vi "PH_Trendviewer_Powermeter.add new result.vi"(0 "i ref in":refnum<vi>, 2 "Energy [J]":dbl, 5 "error in (no error)":errorcluster) -> (14 "i ref out":refnum<vi>, 19 "error out":errorcluster)   [LabVIEW 2014, in "PH_Trendviewer_Powermeter.lvlib"]
doc: "This VI investigates the new incoming data and adds them to the results already collected."
uses:
  PH_Trendviewer_Powermeter.lvlib
  PH_Common/PH_Common.lvlib
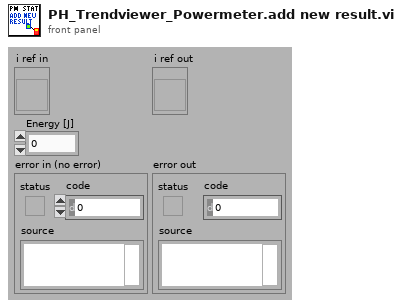
[diagram p1: front panel]
types:
  T1 = cluster{"Time Stamp":timestamp, "Energy [J]":dbl}
  T2 = typedef "PH_Trendviewer_Powermeter.lvlib/PH_Trendviewer_Powermeter.i attribute.ctl" = cluster{"GUI Refs ":cluster{"Status":refnum<vi>, "Result Graph":refnum<vi>, "Mean Data":refnum<vi>, "Std Dev Data":refnum<vi>, "Dummy Mean":refnum<vi>, "Dummy Std Dev":refnum<vi>, "Export Data":refnum<vi>, "Stat or Trend":refnum<vi>, "Delete":refnum<vi>, "Powermeter":refnum<vi>, "Start":refnum<vi>}, "Powermeter":string, "Stat or Trend":bool, "Start":bool, "Data":cluster{"Time Stamp":timestamp, "Energy [J]":dbl}[], "Datasets strored":i32, "Dataarray Size":i32}
  T3 = cluster{"Time Stamp":timestamp, "Energy [J]":dbl}[]
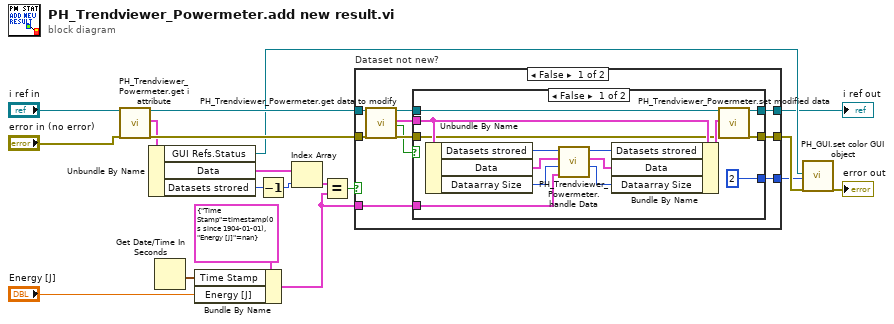
[diagram p0: block diagram]
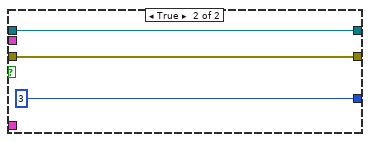
[diagram p2: hidden frame]
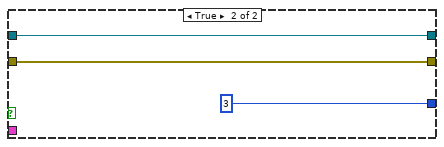
[diagram p3: hidden frame]
diagram:
  n1 = call "PH_Trendviewer_Powermeter.get i attribute.vi"("i ref in"="i ref in", "error in (no error)"="error in (no error)") -> ("i ref out"=w15:refnum<vi>, "i attribute"=w14:T2, "error out"=w16:errorcluster)  [unwired: 15 in]
  n2 = Unbundle By Name(w14) -> ("GUI Refs.Status"=w12:refnum<vi>, "Data"=w8:T3, "Datasets strored"=w6:i32)
  n3 = Get Date/Time In Seconds() -> (seconds since 1Jan1904=w18:timestamp)
  n4 = Bundle By Name(cluster=T1 {"Time Stamp"=timestamp(0 s since 1904-01-01), "Energy [J]"=nan} ("Dataset"), "Time Stamp"=w18, "Energy [J]"="Energy [J]") -> (w1:T1)
  n5 = Decrement(x=w6) -> (x-1=w9:i32)
  n6 = Index Array(array=w8, index=w9) -> (element=w10:T1)
  n7 = Equal?(x=w10, y=w1) -> (x = y?=w7:bool)
  n8 = case "Dataset not new?" shown="False" w7 {
    tunnel: [w26 w49] -> w3
    tunnel: w16 -> [w24 w48]
    tunnel: w15 -> [w23 w49]
    tunnel: [w22 w48] -> w13
    tunnel: [w21 3 ("status")] -> w11
    tunnel: w1 -> [w20 _]
    frame False {
      n9 = call "PH_Trendviewer_Powermeter.get data to modify.vi"("i ref in"=w23, "error in (no error)"=w24) -> ("i ref out"=w27:refnum<vi>, "i attribute"=w29:T2, "timed out"=w25:bool, "error out"=w28:errorcluster)  [unwired: 14 in]
      n10 = case shown="False" w25 {
        tunnel: w29 -> [w37 _]
        tunnel: w28 -> [w36 w45]
        tunnel: [w43 w45] -> w22
        tunnel: w27 -> [w42 w46]
        tunnel: [w41 w46] -> w26
        tunnel: w20 -> [w30 _]
        tunnel: [2 ("status") 3] -> w21
        frame False {
          n11 = Unbundle By Name(w37) -> ("Datasets strored"=w32:i32, "Data"=w31:T3, "Dataarray Size"=w40:i32)
          n12 = call "PH_Trendviewer_Powermeter.handle Data.vi"("New Powermeter Dataset"=w30, "Dataarray Size in"=w40, "Data in"=w31, "Datasets strored in"=w32) -> ("Dataarray Size out"=w38:i32, "Data out"=w33:T3, "Datasets strored out"=w34:i32)  [unwired: 3 in]
          n13 = Bundle By Name(cluster=w37, "Datasets strored"=w34, "Data"=w33, "Dataarray Size"=w38) -> (w39:T2)
          n14 = call "PH_Trendviewer_Powermeter.set modified data.vi"("i ref in"=w42, "i attribute"=w39, "error in (no error)"=w36) -> ("i ref out"=w41:refnum<vi>, "error out"=w43:errorcluster)  [unwired: 15 in]
        }
        frame True {
        }
      }
    }
    frame True {
    }
  }
  "i ref out" <- w3
  n15 = call "PH_GUI.set color GUI object.vi"("GUI object Ref"=w12, "State"=w11, "error in (no error)"=w13) -> ("error out"=→"error out":errorcluster)  [unwired: 16 in]
